vi "Test Reconnect.vi"() -> ()   [LabVIEW 2012]
uses:
  <vilib>/Instr/_visa.llb/VISA Find Search Mode.ctl
  Type Defs/Comm Settings.ctl
panel:
  out "Numeric":i32
  out "read string":string="Ver. 0.1, Feb 10 2013, 23:27:07\r\n"
  out "Selected Port":refnum<visa-resource-name>
  in  "stop":bool
  out "error out":errorcluster
  out "Port List":string[](array[string])
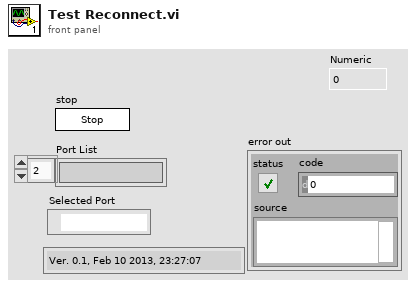
[diagram p1: front panel]
types:
  T1 = typedef "Comm Settings.ctl" = cluster{"Port":refnum<visa-resource-name>, "Baud Rate":u32, "Data Bits":u16, "Parity":u16, "Stop Bits":u16, "Flow Control":u16}
  T2 = typedef "VISA Find Search Mode.ctl" = u32
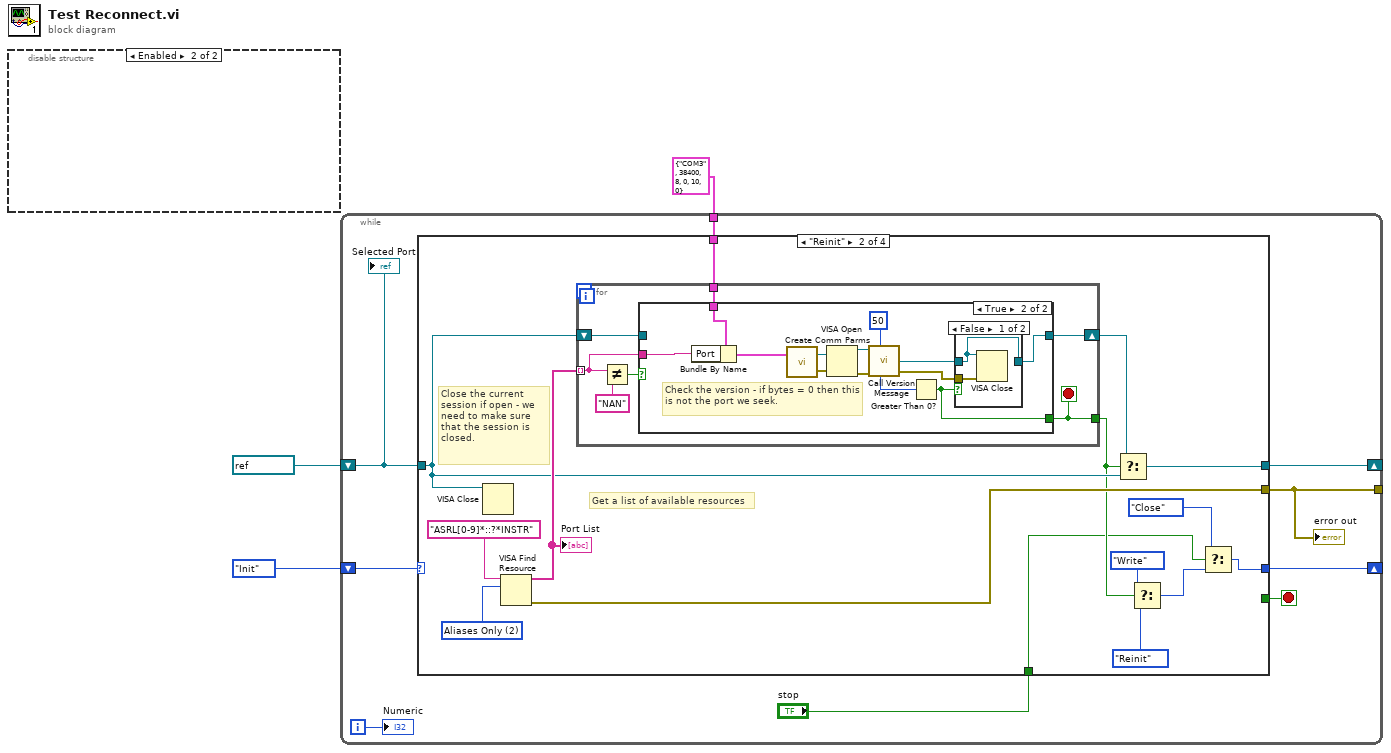
[diagram p0: block diagram]
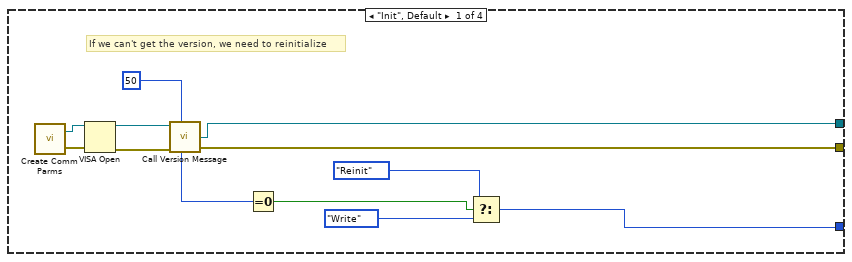
[diagram p3: hidden frame]
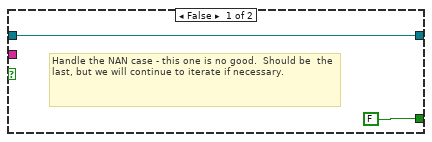
[diagram p4: hidden frame]
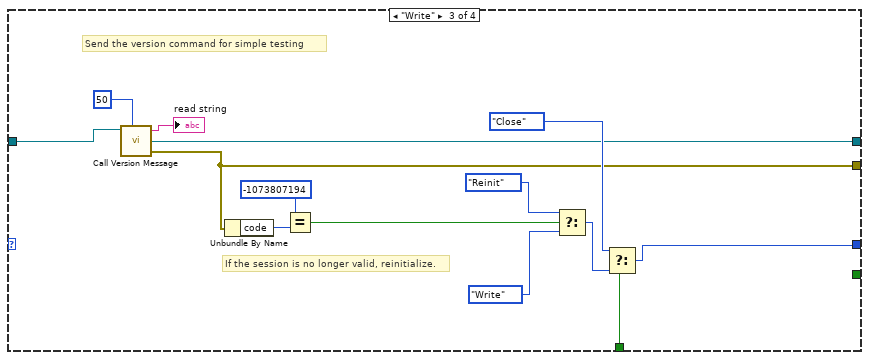
[diagram p6: hidden frame]
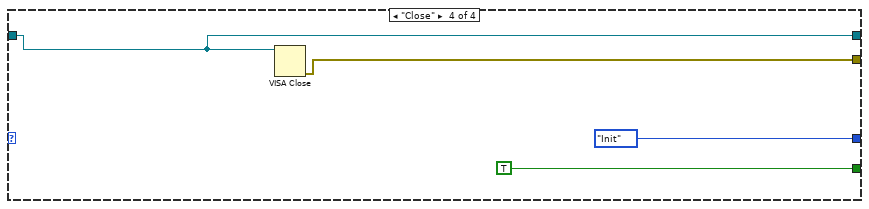
[diagram p7: hidden frame]
diagram:
  n1 = disable-structure shown="Enabled" {
    frame Disabled {
    }
    frame Enabled {
    }
  }
  n2 = while {
    tunnel: [w7] -> _
    shift-right: [w11] -> _
    shift-left: refnum<visa-resource-name> "COM3" ("VISA resource name") -> [w12]
    shift-right: [w9] -> _
    shift-left: enum16{"Reinit", "Init", "Write", "Close"}."Init" -> [w10]
    tunnel: T1 {"Port"="COM3", "Baud Rate"=38400, "Data Bits"=8, "Parity"=0, "Stop Bits"=10, "Flow Control"=0} ("Com Parms") -> [w6]
    i -> [w4]
    stop <- w8 stop-if-true
    n3 = case shown="\"Reinit\"" w10 {
      tunnel: w12 -> [_ w32 w68 w82]
      tunnel: [w17 w35 w67 w82] -> w11
      tunnel: [w18 w34 w70 w81] -> w7
      tunnel: [w22 w26 w75 enum16{"Reinit", "Init", "Write", "Close"}."Init"] -> w9
      tunnel: [_ _ _ TRUE] -> w8
      tunnel: w6 -> [_ w29 _ _]
      tunnel: "stop" -> [_ w25 w65 _]
      frame "Init", Default {
        # "If we can't get the version, we need to reinitialize"
        n4 = call "Create Comm Parms.vi"() -> ("error out"=w15:errorcluster, "VISA resource name out"=w16:refnum<visa-resource-name>)  [unwired: 2 in]
        n5 = VISA Open(error in (no error)=w15, VISA resource name=w16) -> (VISA resource name=w20:refnum<visa-resource-name>, error out=w19:errorcluster)  [unwired: 3 in]
        n6 = call "Call Version Message.vi"("VISA resource name out"=w20, "delay before read (ms)"=u32 50, "error in"=w19) -> ("bytes read"=w14:u32, "VISA resource name out 2"=w17:refnum<visa-resource-name>, "error out"=w18:errorcluster)  [unwired: 2 in, 1 out]
        n7 = Equal To 0?(x=w14) -> (x = 0?=w13:bool)
        n8 = Select(t=enum16{"Reinit", "Init", "Write", "Close"}."Reinit", s=w13, f=enum16{"Reinit", "Init", "Write", "Close"}."Write") -> (s? t:f=w22:enum16{"Reinit", "Init", "Write", "Close"})
      }
      frame "Reinit" {
        w39 = T2 2 items=["Canonical Names Only"=0, "Aliases Only"=2, "Include Matching Aliases"=3, "Include All Aliases"=4] ("Search Mode")
        # "Close the current session if open - we need to make sure that the session is closed."
        # "Get a list of available resources"
        n9 = VISA Close(VISA resource name=w32) -> ()  [unwired: 1 in, 1 out]
        n10 = VISA Find Resource(10:w39, 11:"ASRL[0-9]*::?*INSTR" ("expression (\"?*\")")) -> (0:w34:errorcluster, 3:w33:string[])  [unwired: 1 in, 1 out]
        "Port List" <- w33
        n11 = for {
          tunnel: w33 -> [w44] mode=indexing
          shift-right: [w43] -> w31
          shift-left: w32 -> [w42]
          tunnel: [w41] -> w30
          tunnel: w29 -> [w40]
          stop <- w41 stop-if-true
          n12 = Not Equal?(x=w44, y="NAN" ("x")) -> (x != y?=w45:bool)
          n13 = case shown="True" w45 {
            tunnel: w44 -> [_ w49]
            tunnel: [w48 w54] -> w43
            tunnel: w42 -> [w48 _]
            tunnel: [FALSE w57] -> w41
            tunnel: w40 -> [_ w53]
            frame False {
              # "Handle the NAN case - this one is no good.  Should be  the last, but we will continue to iterate if necessary."
            }
            frame True {
              # "Check the version - if bytes = 0 then this is not the port we seek."
              n14 = Bundle By Name(cluster=w53, "Port"=w49) -> (w52:T1)
              n15 = call "Create Comm Parms.vi"(3:w52) -> ("error out"=w50:errorcluster, "VISA resource name out"=w51:refnum<visa-resource-name>)  [unwired: 1 in]
              n16 = VISA Open(error in (no error)=w50, VISA resource name=w51) -> (VISA resource name=w60:refnum<visa-resource-name>, error out=w59:errorcluster)  [unwired: 3 in]
              n17 = call "Call Version Message.vi"("VISA resource name out"=w60, "delay before read (ms)"=u32 50, "error in"=w59) -> ("bytes read"=w58:u32, "VISA resource name out 2"=w56:refnum<visa-resource-name>, "error out"=w55:errorcluster)  [unwired: 2 in, 1 out]
              n18 = Greater Than 0?(x=w58) -> (x > 0?=w57:bool)
              n19 = case shown="False" w57 {
                tunnel: w56 -> [w62 w64]
                tunnel: w55 -> [w63 _]
                tunnel: [w62 w64] -> w54
                frame False {
                  n20 = VISA Close(VISA resource name=w62, error in (no error)=w63) -> ()  [unwired: 1 out]
                }
                frame True {
                }
              }
            }
          }
        }
        n21 = Select(t=w31, s=w30, f=w32) -> (s? t:f=w35:refnum<visa-resource-name>)
        n22 = Select(t=enum16{"Reinit", "Init", "Write", "Close"}."Write", s=w30, f=enum16{"Reinit", "Init", "Write", "Close"}."Reinit") -> (s? t:f=w28:enum16{"Reinit", "Init", "Write", "Close"})
        n23 = Select(t=enum16{"Reinit", "Init", "Write", "Close"}."Close", s=w25, f=w28) -> (s? t:f=w26:enum16{"Reinit", "Init", "Write", "Close"})
      }
      frame "Write" {
        # "If the session is no longer valid, reinitialize."
        # "Send the version command for simple testing"
        n24 = call "Call Version Message.vi"("VISA resource name out"=w68, "delay before read (ms)"=u32 50) -> ("read string"=→"read string":string, "VISA resource name out 2"=w67:refnum<visa-resource-name>, "error out"=w70:errorcluster)  [unwired: 3 in, 1 out]
        n25 = Unbundle By Name(w70) -> ("code"=w71:i32)
        n26 = Equal?(x=-1073807194, y=w71) -> (x = y?=w77:bool)
        n27 = Select(t=enum16{"Reinit", "Init", "Write", "Close"}."Reinit", s=w77, f=enum16{"Reinit", "Init", "Write", "Close"}."Write") -> (s? t:f=w76:enum16{"Reinit", "Init", "Write", "Close"})
        n28 = Select(t=enum16{"Reinit", "Init", "Write", "Close"}."Close", s=w65, f=w76) -> (s? t:f=w75:enum16{"Reinit", "Init", "Write", "Close"})
      }
      frame "Close" {
        n29 = VISA Close(VISA resource name=w82) -> (error out=w81:errorcluster)  [unwired: 1 in]
      }
    }
    "error out" <- w7
    "Selected Port" <- w12
    "Numeric" <- w4
  }
